vi "Initialize Axes.vi"(8 "error in (no error)":errorcluster, 11 "Port In":T1={"P type"=1, "VISA resource name out"="", " Terminator"="\n\r", "Timeout"=300} {"Timeout" step=10; "P type" items=["none", "RS-232C", "IEEE-488.1", "IEEE-488.2"]}) -> (0 "error out":errorcluster, 3 "Port Out":T1)   [LabVIEW 2021]
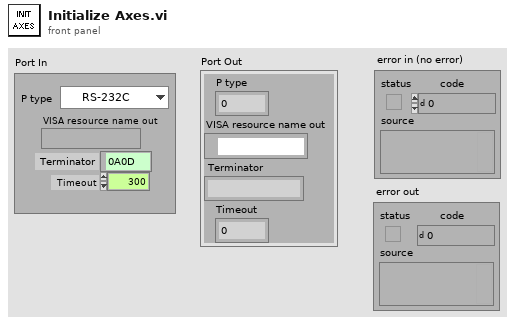
[diagram p1: front panel]
types:
  T1 = cluster{"P type":u16, "VISA resource name out":refnum<visa-resource-name>, " Terminator":string, "Timeout":i32}
  T2 = cluster{"P type":u16, "reference":refnum<visa-resource-name>, " Terminator ":string, "Timeout":i32}
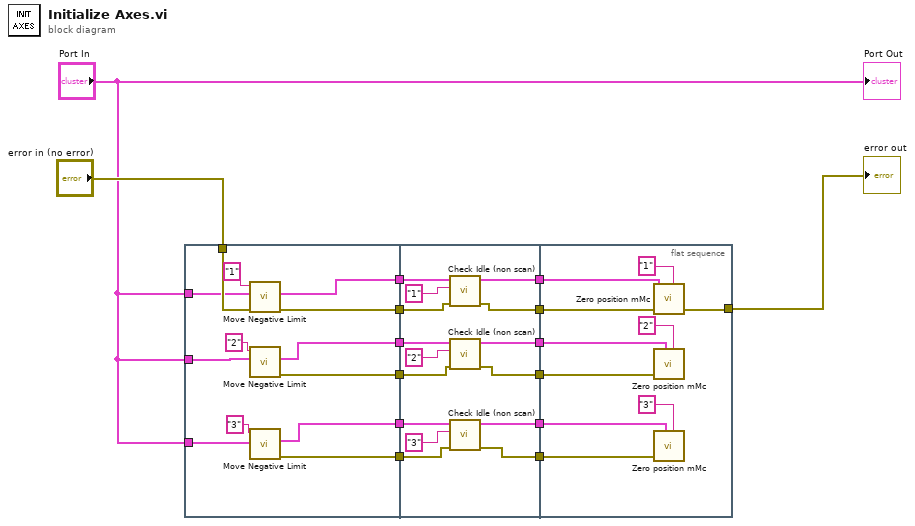
[diagram p0: block diagram]
diagram:
  n1 = flat-sequence {
    tunnel: "error in (no error)" -> [w28]
    tunnel: "Port In" -> [w27]
    tunnel: [w26] -> w13
    tunnel: [w25] -> w11
    tunnel: "Port In" -> [w24]
    tunnel: [w23] -> w9
    tunnel: "Port In" -> [w22]
    tunnel: [w21] -> w6
    tunnel: [w19] -> w5
    tunnel: [w18] -> w3
    tunnel: [w34] -> w14
    tunnel: w13 -> [w33]
    tunnel: [w31] -> w12
    tunnel: w11 -> [w32]
    tunnel: [w38] -> w10
    tunnel: w9 -> [w39]
    tunnel: [w29] -> w7
    tunnel: w6 -> [w43]
    tunnel: w5 -> [w37]
    tunnel: [w36] -> w4
    tunnel: w3 -> [w42]
    tunnel: [w41] -> w2
    tunnel: w14 -> [w53]
    tunnel: w12 -> [w52]
    tunnel: w10 -> [w51]
    tunnel: w7 -> [w50]
    tunnel: w4 -> [w48]
    tunnel: w2 -> [w47]
    tunnel: [w44] -> w1
    frame #0 {
      n2 = call "Move Negative Limit.vi"("error in (no error)"=w28, "Port In"=w27, "Controller #"="1") -> ("error out"=w25:errorcluster, "Port Out"=w26:T1)  [unwired: 7 in]
      n3 = call "Move Negative Limit.vi"("Port In"=w24, "Controller #"="2") -> ("error out"=w23:errorcluster, "Port Out"=w19:T1)  [unwired: 8 in]
      n4 = call "Move Negative Limit.vi"("Port In"=w22, "Controller #"="3") -> ("error out"=w21:errorcluster, "Port Out"=w18:T1)  [unwired: 8 in]
    }
    frame #1 {
      n5 = call "Check Idle (non scan).vi"("error in (no error)"=w32, "Controller #"="1", "Port In"=w33) -> ("error out (no error)"=w31:errorcluster, "Port Out"=w34:T2)  [unwired: 7 in]
      n6 = call "Check Idle (non scan).vi"("error in (no error)"=w39, "Controller #"="2", "Port In"=w37) -> ("error out (no error)"=w38:errorcluster, "Port Out"=w36:T2)  [unwired: 7 in]
      n7 = call "Check Idle (non scan).vi"("error in (no error)"=w43, "Controller #"="3", "Port In"=w42) -> ("error out (no error)"=w29:errorcluster, "Port Out"=w41:T2)  [unwired: 7 in]
    }
    frame #2 {
      n8 = call "Zero position mMc.vi"("Port"=w53, "error in (no error)"=w52, "Controller #"="1") -> ("error out"=w44:errorcluster)  [unwired: 6 in]
      n9 = call "Zero position mMc.vi"("Port"=w48, "error in (no error)"=w51, "Controller #"="2") -> ()  [unwired: 6 in, 1 out]
      n10 = call "Zero position mMc.vi"("Port"=w47, "error in (no error)"=w50, "Controller #"="3") -> ()  [unwired: 6 in, 1 out]
    }
  }
  "error out" <- w1
  "Port Out" <- "Port In"
